vi "Main.vi"(11 "Module Admin":refnum<class "Delacor_lib_QMH_Module Admin.lvclass">) -> ()   [LabVIEW 2020, in "Acquisition.lvlib"]
doc: "This template is based off of the Queued Message Handler design pattern and the Queued Message Handler project template that ships with LabVIEW.\n\nThe main difference is that the queue is private to this module and communication between modules is performed via Broadcast and Request events.\n\nRequest events are wrapped in public API methods and are handled in the Event Handling Loop (EHL) of this VI. Any module can register for Broadcast events sent by this module. The EHL generates messages based on user interface actions.\n\nThe Message Handling Loop (MHL) processes messages generated by the EHL, or by other messages. The messages are string values, so new messages can be added easily to the Message Cases case structure in the MHL. Each message cluster can also provide an optional value for Message Data, which is a variant that can be converted to whatever message-specific data is required.\n_____\nBased on Delacor QMH Project Template 5.0.0.82."
uses:
  Acquisition.lvlib
  <vilib>/Delacor/Delacor QMH/Libraries/Module Admin_class/Delacor_lib_QMH_Module Admin.lvclass
  Module Data--cluster.ctl
  Stop Helper Loop Argument--cluster.ctl
  <vilib>/Delacor/Delacor QMH/Libraries/Message Queue_class/Delacor_lib_QMH_Message Queue.lvclass/Delacor_lib_QMH_Message Queue.ctl
  Stop Argument--cluster.ctl
  <vilib>/Delacor/Delacor QMH/Libraries/Module Admin_class/Delacor_lib_QMH_Module Admin.lvclass/Delacor_lib_QMH_Module Admin.ctl
  <vilib>/Utility/miscctls.llb/LVPointTypeDef.ctl
  <vilib>/Delacor/Delacor QMH/Libraries/Message Queue_class/Delacor_lib_QMH_Enqueue Message (Single).vi
  <vilib>/Delacor/Delacor QMH/Libraries/Module Admin_class/Delacor_lib_QMH_Get External Launch.vi
  <vilib>/Utility/error.llb/Error Cluster From Error Code.vi
  <vilib>/ErrorRing/Error Ring.xnode
  <vilib>/Delacor/Delacor QMH/Libraries/Message Queue_class/Delacor_lib_QMH_Message Queue.lvclass
panel:
  out "Time Stamp":timestamp
  in  "Simulate MHL Error":bool
  in  "Simulate EHL Error":bool
  out "error out":errorcluster
  out "Status":string
  # "Other QMH Modules communicate with this Module via its Public API (wrappers for its Request Events).\n\nThis Module communicates with other Modules via its Broadcast Events.\nAny module that wants to get these messages, just registers for this module's Broadcast events."
  # "This template is for the Delacor Modified Queued Message Handler design pattern.\n\nSee the block diagram for more information on how to use this template."
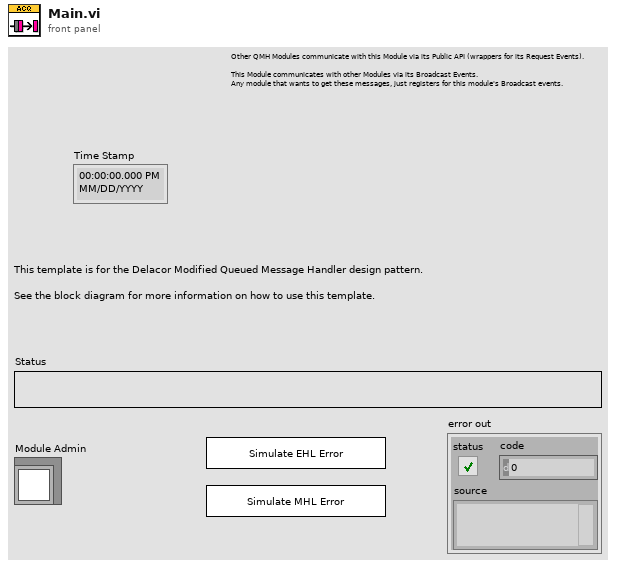
[diagram p1: front panel]
types:
  T1 = typedef "Acquisition.lvlib/Request Events--cluster.ctl" = cluster{"Stop Module":refnum<user-event>, "Show Panel":refnum<user-event>, "Hide Panel":refnum<user-event>, "Get Module Execution Status":refnum<user-event>, "Show Diagram":refnum<user-event>, "Start Helper Loop":refnum<user-event>, "Stop Helper Loop":refnum<user-event>}
  T2 = typedef "Acquisition.lvlib/Module Data--cluster.ctl" = cluster{"Status":string}
  T3 = enum32{"invalid lock state", "Not Locked", "Locked (No Password)", "Password-protected"}
  T4 = typedef "Acquisition.lvlib/Stop Argument--cluster.ctl" = cluster{"Origin":string, "Exit via Stop Module Req?":bool, "Wait for Module to stop?":bool}
  T5 = typedef "LVPointTypeDef.ctl" = cluster{"Horizontal":i16, "Vertical":i16}
  T6 = enum32{"Invalid", "Standard", "Closed", "Hidden", "Minimized", "Maximized"}
  T7 = typedef "Acquisition.lvlib/Stop Helper Loop Argument--cluster.ctl" = cluster{"Boolean":bool}
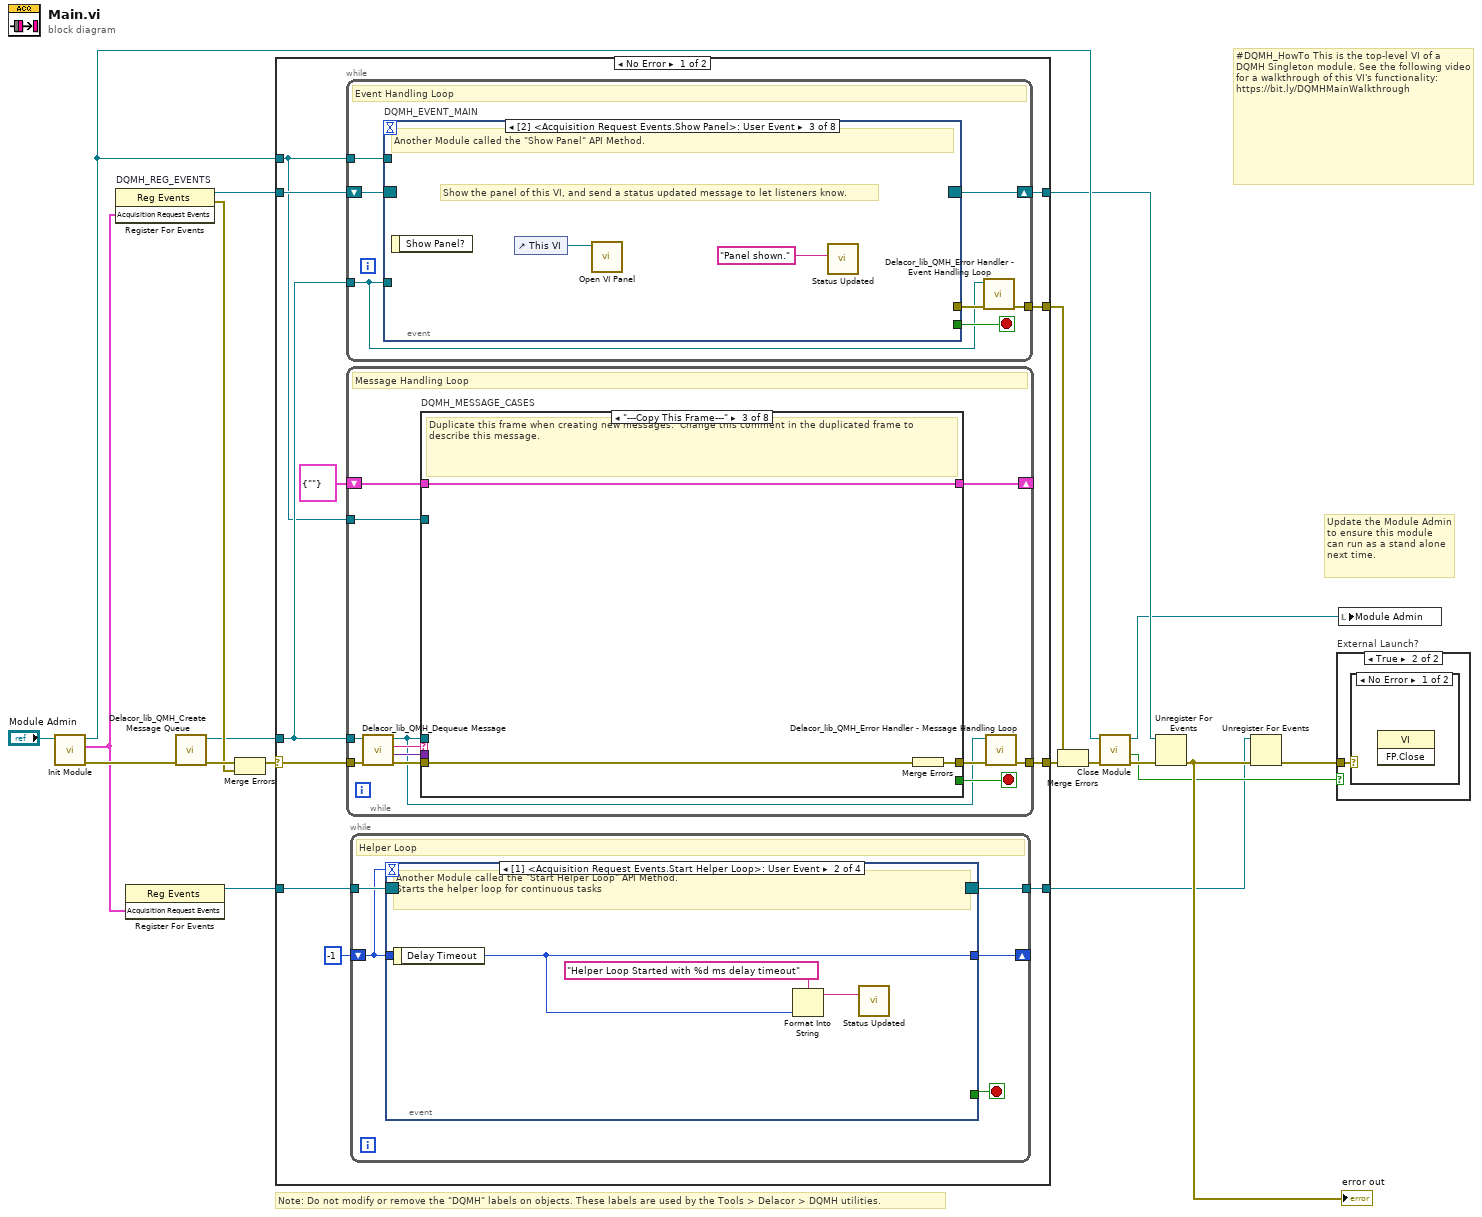
[diagram p0: block diagram]
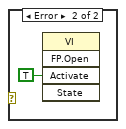
[diagram p3: hidden frame]
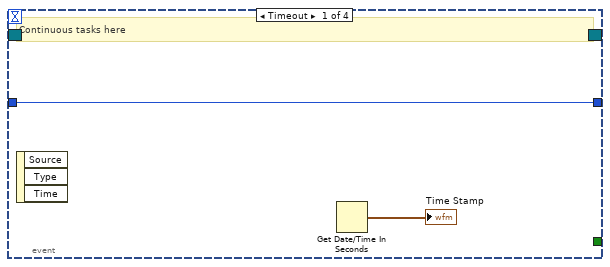
[diagram p4: hidden frame]
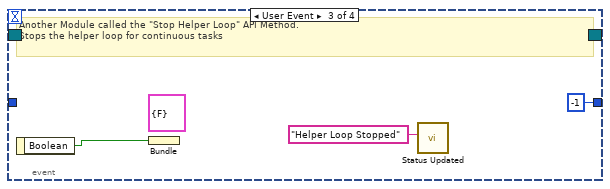
[diagram p5: hidden frame]
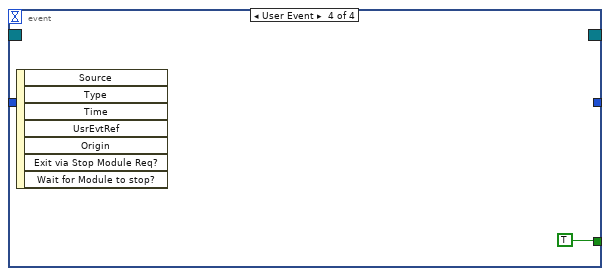
[diagram p6: hidden frame]
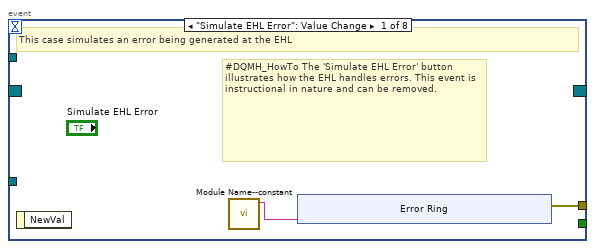
[diagram p7: hidden frame]
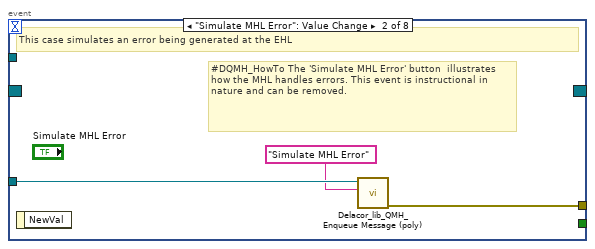
[diagram p8: hidden frame]
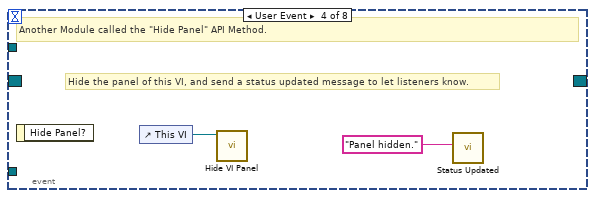
[diagram p9: hidden frame]
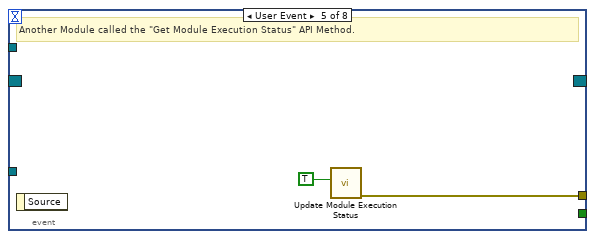
[diagram p10: hidden frame]
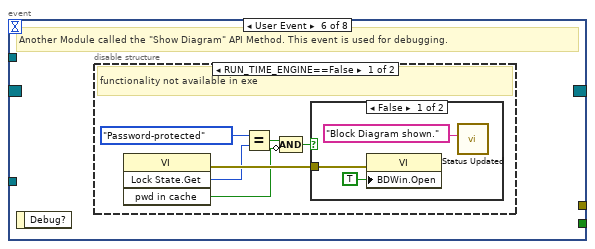
[diagram p11: hidden frame]
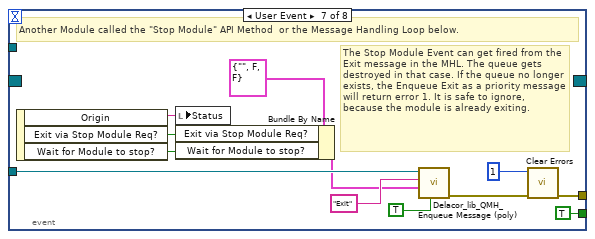
[diagram p14: hidden frame]
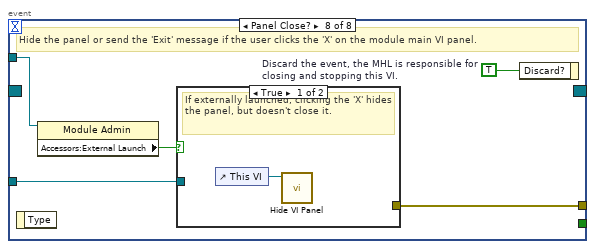
[diagram p15: hidden frame]
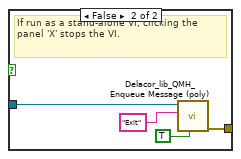
[diagram p16: hidden frame]
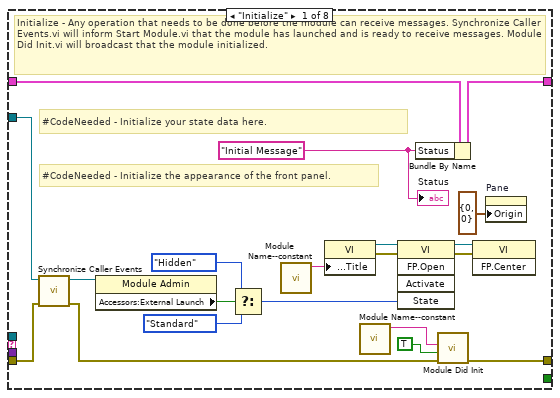
[diagram p17: hidden frame]
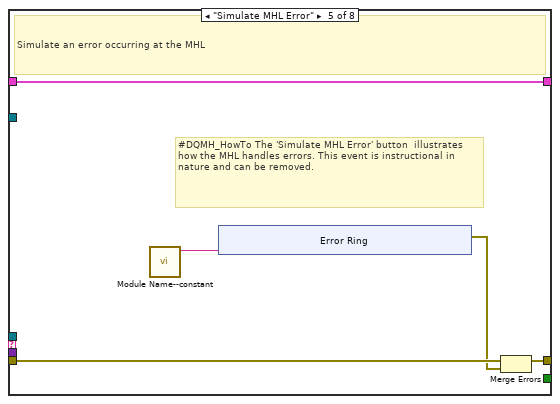
[diagram p20: hidden frame]
diagram:
  # "#DQMH_HowTo This is the top-level VI of a DQMH Singleton module. See the following video for a walkthrough of this VI's functionality: https://bit.ly/DQMHMainWalkthrough"
  # "Note: Do not modify or remove the \"DQMH\" labels on objects. These labels are used by the Tools > Delacor > DQMH utilities."
  # "Update the Module Admin to ensure this module can run as a stand alone next time."
  n1 = call "Init Module.vi"("Singleton Module Admin in"="Module Admin") -> ("error out"=w19:errorcluster, "Acquisition Request Events"=w3:T1, "Singleton Module Admin out"=w11:refnum<class "Delacor_lib_QMH_Module Admin.lvclass">)  [unwired: 8 in]
  n2 = register-events "DQMH_REG_EVENTS"(w3) -> (reference out=w9:refnum<event-registration>, error out=w12:errorcluster)  [unwired: 2 in]
  n3 = register-events(w3) -> (reference out=w4:refnum<event-registration>)  [unwired: 2 in, 1 out]
  n4 = call <vilib>:"Delacor_lib_QMH_Create Message Queue.vi"("error in (no error)"=w19) -> ("error out"=w14:errorcluster, "Message Queue"=w8:refnum<class "Delacor_lib_QMH_Message Queue.lvclass">)  [unwired: 9 in]
  n5 = Merge Errors(w14, w12) -> (w13:errorcluster)
  n6 = case shown="No Error" w13 {
    selector: w13 -> [w29 w202]
    tunnel: [w31 w201] -> w20
    tunnel: [w28 w207] -> w10
    tunnel: w9 -> [w26 w207]
    tunnel: w8 -> [w25 w200]
    tunnel: [w30 _] -> w17
    tunnel: w11 -> [w24 w203]
    tunnel: w4 -> [w23 w199]
    tunnel: [w22 w199] -> w1
    frame No Error {
      n7 = while {
        tunnel: w25 -> [w46]
        shift-right: [w49] -> w28
        shift-left: w26 -> [w50]
        tunnel: [w51] -> w30
        tunnel: w24 -> [w47]
        stop <- w48 stop-if-true
        # "Event Handling Loop"
        n8 = event "DQMH_EVENT_MAIN" shown="[2] <Acquisition Request Events.Show Panel>: User Event" {
          selector: w50 -> [_ _ _ _ _ _ _ _]
          dyn-events: [_ _ _ _ _ _ _ _] -> w49
          timeout: _ -> [_ _ _ _ _ _ _ _]
          tunnel: [_ _ _ _ _ _ TRUE ("Discard?") _] -> w48
          tunnel: w46 -> [_ w63 _ _ _ _ w87 w94]
          tunnel: [w54 w64 _ _ w70 _ w90 w96] -> w52
          tunnel: w47 -> [_ _ _ _ _ _ _ w93]
          event "Simulate EHL Error": Value Change {
            # "#DQMH_HowTo The 'Simulate EHL Error' button  illustrates how the EHL handles errors. This event is instructional in nature and can be removed."
            # "This case simulates an error being generated at the EHL"
            n9 = event-data() -> ()  [unwired: 1 in, 1 out]
            n10 = call "Module Name--constant.vi"() -> ("Module Name"=w53:string)  [unwired: 11 in]
            n11 = xnode "Error Ring"("parameter 0"=w53) -> ("error out"=w54:errorcluster)
          }
          event "Simulate MHL Error": Value Change {
            # "#DQMH_HowTo The 'Simulate MHL Error' button  illustrates how the MHL handles errors. This event is instructional in nature and can be removed."
            # "This case simulates an error being generated at the EHL"
            n12 = event-data() -> ()  [unwired: 1 in, 1 out]
            n13 = call-poly <vilib>:"Delacor_lib_QMH_Enqueue Message (poly).vi"("Message"="Simulate MHL Error", "Message Queue in"=w63) -> ("error out"=w64:errorcluster)  [unwired: 8 in, 1 out]
          }
          event User Event {
            # "Show the panel of this VI, and send a status updated message to let listeners know."
            # "Another Module called the \"Show Panel\" API Method."
            n14 = event-data() -> ()  [unwired: 1 in, 1 out]
            n15 = control-ref of="This VI"() -> (w66:refnum<vi>)
            n16 = call "Open VI Panel.vi"("VI"=w66) -> ()  [unwired: 10 in, 1 out]
            n17 = call "Status Updated.vi"("Status"="Panel shown." ("format string")) -> ()  [unwired: 10 in, 1 out]
          }
          event User Event {
            # "Hide the panel of this VI, and send a status updated message to let listeners know."
            # "Another Module called the \"Hide Panel\" API Method."
            n18 = event-data() -> ()  [unwired: 1 in, 1 out]
            n19 = control-ref of="This VI"() -> (w68:refnum<vi>)
            n20 = call "Hide VI Panel.vi"("VI"=w68) -> ()  [unwired: 10 in, 1 out]
            n21 = call "Status Updated.vi"("Status"="Panel hidden." ("format string")) -> ()  [unwired: 10 in, 1 out]
          }
          event User Event {
            # "Another Module called the \"Get Module Execution Status\" API Method."
            n22 = event-data() -> ()  [unwired: 1 in, 1 out]
            n23 = call "Update Module Execution Status.vi"("Running?"=TRUE) -> ("error out"=w70:errorcluster)  [unwired: 10 in]
          }
          event User Event {
            # "Another Module called the \"Show Diagram\" API Method. This event is used for debugging."
            n24 = event-data() -> ()  [unwired: 1 in, 1 out]
            n25 = disable-structure shown="RUN_TIME_ENGINE==False" {
              frame condition #0 (active) {
                # "functionality not available in exe"
                n26 = invoke class="VI" method="Lock State.Get"() -> (error out=w76:errorcluster, "Get Lock State"=w75:T3, "pwd in cache"=w72:bool)  [unwired: 4 in, 1 out]
                n27 = Equal?(x=T3."Password-protected", y=w75) -> (x = y?=w73:bool)
                n28 = Compound Arithmetic op=AND(w73, invert w72) -> (w71:bool)
                n29 = case shown="False" w71 {
                  tunnel: w76 -> [w79 _]
                  frame False {
                    n30 = property class="VI"(error in=w79, "BDWin.Open"=TRUE ("Block Diagram Window:Open")) -> ()  [unwired: 1 in, 2 out]
                    n31 = call "Status Updated.vi"("Status"="Block Diagram shown." ("format string")) -> ()  [unwired: 10 in, 1 out]
                  }
                  frame True {
                    # "Password-protected VI, and the password is not in the cache. Do not show the diagram."
                  }
                }
              }
              frame condition #1 {
              }
            }
          }
          event User Event {
            # "The Stop Module Event can get fired from the Exit message in the MHL. The queue gets destroyed in that case. If the queue no longer exists, the Enqueue Exit as a priority message will return error 1. It is safe to ignore, because the module is already exiting."
            # "Another Module called the \"Stop Module\" API Method  or the Message Handling Loop below."
            n32 = event-data() -> ("Origin"=w86:string, "Exit via Stop Module Req?"=w82:bool, "Wait for Module to stop?"=w81:bool)  [unwired: 1 in]
            n33 = local write "Status"(w86) -> ()
            n34 = Bundle By Name(cluster=T4 {"Origin"="", "Exit via Stop Module Req?"=FALSE, "Wait for Module to stop?"=FALSE} ("Stop Argument"), "Exit via Stop Module Req?"=w82, "Wait for Module to stop?"=w81) -> (w80:T4)
            n35 = call-poly <vilib>:"Delacor_lib_QMH_Enqueue Message (poly).vi"("Priority Message? (F)"=TRUE, "Message Data"=w80, "Message"="Exit", "Message Queue in"=w87) -> ("error out"=w91:errorcluster)  [unwired: 6 in, 1 out]
            n36 = call <vilib>:"Clear Errors.vi"("error in (no error)"=w91, "specific error code to clear (0: all)"=1) -> ("error out"=w90:errorcluster)  [unwired: 4 in, 1 out]
          }
          event Panel Close? {
            w95 = TRUE  # Discard the event, the MHL is responsible for closing and stopping this VI.
            # "Hide the panel or send the 'Exit' message if the user clicks the 'X' on the module main VI panel."
            n37 = event-data() -> ()  [unwired: 1 in, 1 out]
            n38 = property class="Module Admin"(reference=w93) -> ("Accessors:External Launch"=w92:bool)  [unwired: 1 in, 2 out]
            n39 = case shown="True" w92 {
              tunnel: w94 -> [_ w100]
              tunnel: [_ w101] -> w96
              frame True {
                # "If externally launched, clicking the 'X' hides the panel, but doesn't close it."
                n40 = control-ref of="This VI"() -> (w97:refnum<vi>)
                n41 = call "Hide VI Panel.vi"("VI"=w97) -> ()  [unwired: 10 in, 1 out]
              }
              frame False {
                # "If run as a stand-alone VI, clicking the panel 'X' stops the VI."
                n42 = call-poly <vilib>:"Delacor_lib_QMH_Enqueue Message (poly).vi"("Priority Message? (F)"=TRUE, "Message"="Exit", "Message Queue in"=w100) -> ("error out"=w101:errorcluster)  [unwired: 7 in, 1 out]
              }
            }
            n43 = event-data("Discard?"=w95) -> ()  [unwired: 1 in, 1 out]
          }
        }
        n44 = call-dynamic "Delacor_lib_QMH_Error Handler - Event Handling Loop.vi"("error in (no error)"=w52, "Message Queue in"=w46) -> ("dup error in"=w51:errorcluster)  [unwired: 8 in, 1 out]
      }
      n45 = while {
        tunnel: w25 -> [w104]
        shift-right: [w108] -> _
        shift-left: T2 {"Status"=""} ("Data Cluster") -> [w109]
        tunnel: w29 -> [w112]
        tunnel: [w110] -> w31
        tunnel: w24 -> [w102]
        stop <- w107 stop-if-true
        # "Message Handling Loop"
        n46 = call-dynamic "Delacor_lib_QMH_Dequeue Message.vi"("error in (no error)"=w112, "Message Queue in"=w104) -> ("error out"=w111:errorcluster, "Message Data"=w105:variant, "Message"=w106:string, "Message Queue out"=w103:refnum<class "Delacor_lib_QMH_Message Queue.lvclass">)  [unwired: 6 in]
        n47 = case "DQMH_MESSAGE_CASES" shown="\"---Copy This Frame---\"" w106 {
          selector: w106 -> [_ _ _ _ _ _ _ w186]
          tunnel: w103 -> [_ _ _ _ _ w156 w178 _]
          tunnel: w111 -> [w131 w135 w138 w140 w145 w163 w184 w188]
          tunnel: [w129 w135 w137 w140 w144 w159 w181 w189] -> w113
          tunnel: w109 -> [w120 w134 w136 w139 w142 w158 w177 w187]
          tunnel: [w119 w134 w136 w139 w142 w158 w177 w187] -> w108
          tunnel: [_ _ _ _ _ _ w176 _] -> w107
          tunnel: w105 -> [_ _ _ _ _ w157 w175 _]
          tunnel: w102 -> [w121 _ _ _ _ w155 w170 _]
          frame "Initialize" {
            w114 = "Initial Message" ("Initial Message")
            # "#CodeNeeded - Initialize the appearance of the front panel."
            # "#CodeNeeded - Initialize your state data here."
            # "Initialize - Any operation that needs to be done before the module can receive messages. Synchronize Caller Events.vi will inform Start Module.vi that the module has launched and is ready to receive messages. Module Did Init.vi will broadcast that the module initialized."
            n48 = call "Synchronize Caller Events.vi"("error in (no error)"=w131, "Singleton Module Admin in"=w121) -> ("error out"=w130:errorcluster, "Singleton Module Admin out"=w116:refnum<class "Delacor_lib_QMH_Module Admin.lvclass">)  [unwired: 8 in]
            n49 = property class="Module Admin"(reference=w116) -> ("Accessors:External Launch"=w125:bool)  [unwired: 1 in, 2 out]
            n50 = Select(t=T6."Hidden" ("State"), s=w125, f=T6."Standard" ("State")) -> (s? t:f=w122:T6)
            n51 = call "Module Name--constant.vi"() -> ("Module Name"=w128:string)  [unwired: 11 in]
            n52 = property class="VI"("Front Panel.Title"=w128) -> (reference out=w127:refnum<vi>, error out=w133:errorcluster)  [unwired: 2 in]
            n53 = call "Module Name--constant.vi"() -> ("Module Name"=w117:string)  [unwired: 11 in]
            n54 = invoke class="VI" method="FP.Open"(reference=w127, error in=w133, "State"=w122) -> (reference out=w126:refnum<vi>, error out=w132:errorcluster)  [unwired: 2 in, 3 out]
            n55 = Bundle By Name(cluster=w120, "Status"=w114) -> (w119:T2)
            n56 = call "Module Did Init.vi"("error in (no error)"=w130, "Initialized?"=TRUE, "Origin"=w117) -> ("error out"=w129:errorcluster)  [unwired: 8 in]
            n57 = invoke class="VI" method="FP.Center"(reference=w126, error in=w132) -> ()  [unwired: 1 in, 3 out]
            n58 = property on="Pane" class="Pane"("Origin"=T5 {"Horizontal"=0, "Vertical"=0}) -> ()  [unwired: 2 in, 2 out]
            "Status" <- w114
          }
          frame "--- Module Specific ---" {
            # "Separator -- The following cases handle messages specific to this Module."
          }
          frame "---Copy This Frame---" {
            # "Duplicate this frame when creating new messages.  Change this comment in the duplicated frame to describe this message."
            n59 = Merge Errors(w138) -> (w137:errorcluster)
          }
          frame "--- Exit and Error Handling---" {
            # "Separator - The following cases handle errors and exit messages."
          }
          frame "Simulate MHL Error" {
            # "#DQMH_HowTo The 'Simulate MHL Error' button  illustrates how the MHL handles errors. This event is instructional in nature and can be removed."
            # "Simulate an error occurring at the MHL"
            n60 = call "Module Name--constant.vi"() -> ("Module Name"=w141:string)  [unwired: 11 in]
            n61 = xnode "Error Ring"("parameter 0"=w141) -> ("error out"=w143:errorcluster)
            n62 = Merge Errors(w145, w143) -> (w144:errorcluster)
          }
          frame "Error" {
            # "#CodeRecommended - If you ever change the name of this \"Error\" message, you'll need to update the name in the Check Loop Error.vi as well."
            # "#CodeRecommended - If the module is running in standalone mode (External Launch = FALSE), this code will pop up an error dialog and call the 'Exit' message if an error occurs. Add more fine-grained error handling here."
            # "Error - Check the error message data and respond accordingly. This message is sent by the \"Error Handler\" VIs at the end of each loop in this application."
            n63 = property class="Module Admin"(reference=w155) -> ("Accessors:External Launch"=w154:bool)  [unwired: 1 in, 2 out]
            n64 = Variant To Data(error in=w163, type=errorcluster {"status"=FALSE, "code"=0, "source"=""} ("error constant"), Variant=w157) -> (data=w164:errorcluster, error out=w161:errorcluster)
            n65 = call "Module Name--constant.vi"() -> ("Module Name"=w153:string)  [unwired: 11 in]
            n66 = call "Error Reported.vi"("Additional Information"=w153, "Error"=w164) -> ()  [unwired: 9 in, 1 out]
            n67 = case shown="False" w154 {
              tunnel: [w169 _] -> w160
              tunnel: w156 -> [w167 _]
              tunnel: w164 -> [w168 _]
              frame False {
                # "If the module is running standalone, then pop up an error dialog and call the \"Exit\" message."
                n68 = call <vilib>:"Simple Error Handler.vi"("error in (no error)"=w168) -> ()  [unwired: 4 in, 5 out]
                n69 = call-poly <vilib>:"Delacor_lib_QMH_Enqueue Message (poly).vi"("Priority Message? (F)"=TRUE, "Message"="Exit", "Message Queue in"=w167) -> ("error out"=w169:errorcluster)  [unwired: 7 in, 1 out]
              }
              frame True {
                # "If the module was launched externally, calling the Error Reported broadcast VI is the only action performed by the \"Error\" message. The module's caller can then process the error appropriately."
              }
            }
            n70 = Merge Errors(w161, w160) -> (w159:errorcluster)
            n71 = local write "error out"(w159) -> ()
          }
          frame "Exit" {
            w174 = 91  # 91: not all Exit messages will have an argument
            w176 = TRUE  # Stop the VI
            # "Release the message queue reference"
            # "#CodeNeeded - Add any required cleanup code here"
            # "Exit - Exit the application."
            n72 = Variant To Data(error in=w184, type=T4 {"Origin"="", "Exit via Stop Module Req?"=FALSE, "Wait for Module to stop?"=FALSE} ("Stop Argument"), Variant=w175) -> (data=w172:T4, error out=w180:errorcluster)
            n73 = call <vilib>:"Clear Errors.vi"("error in (no error)"=w180, "specific error code to clear (0: all)"=w174) -> ("error out"=w183:errorcluster)  [unwired: 4 in, 1 out]
            n74 = control-ref of="This VI"() -> (w171:refnum<vi>)
            n75 = call-dynamic "Delacor_lib_QMH_Release Message Queue.vi"("error in (no error)"=w183, "Message Queue"=w178) -> ("error out"=w182:errorcluster)  [unwired: 9 in]
            n76 = call "Handle Exit.vi"("Stop Argument"=w172, "Admin in"=w170, "VI reference"=w171) -> ("error out"=w179:errorcluster)  [unwired: 7 in, 1 out]
            n77 = Merge Errors(w182, w179) -> (w181:errorcluster)
          }
          frame Default {
            # "'Default' case only runs if there is a message that isn't defined in any of the other cases.  Output a programming error."
            n78 = call "Module Name--constant.vi"() -> ("Module Name"=w185:string)  [unwired: 11 in]
            n79 = xnode "Error Ring"("parameter 0"=w186, "parameter 1"=w185) -> ("error out"=w190:errorcluster)
            n80 = Merge Errors(w188, w190) -> (w189:errorcluster)
          }
        }
        n81 = call-dynamic "Delacor_lib_QMH_Error Handler - Message Handling Loop.vi"("error in (no error)"=w113, "Message Queue in"=w103) -> ("dup error in"=w110:errorcluster)  [unwired: 8 in, 1 out]
      }
      n82 = while {
        tunnel: w23 -> [w36]
        tunnel: [w35] -> w22
        shift-right: [w33] -> _
        shift-left: -1 -> [w32]
        stop <- w34 stop-if-true
        # "Helper Loop"
        n83 = event shown="[1] <Acquisition Request Events.Start Helper Loop>: User Event" {
          selector: w36 -> [_ _ _ _]
          dyn-events: [_ _ _ _] -> w35
          timeout: w32 -> [_ _ _ _]
          tunnel: [_ _ _ TRUE] -> w34
          tunnel: [w38 w41 -1 _] -> w33
          tunnel: w32 -> [w38 _ _ _]
          event Timeout {
            # "Continuous tasks here"
            n84 = event-data() -> ()  [unwired: 1 in, 3 out]
            n85 = Get Date/Time In Seconds() -> (seconds since 1Jan1904=→"Time Stamp":timestamp)
          }
          event User Event {
            # "Another Module called the \"Start Helper Loop\" API Method.\nStarts the helper loop for continuous tasks"
            n86 = event-data() -> ("Delay Timeout"=w41:i32)  [unwired: 1 in]
            n87 = Format Into String(format string="Helper Loop Started with %d ms delay timeout", w41) -> (resulting string=w40:string)  [unwired: 2 in, 1 out]
            n88 = call "Status Updated.vi"("Status"=w40) -> ()  [unwired: 10 in, 1 out]
          }
          event User Event {
            (unwired) T7 {"Boolean"=FALSE} ("Stop Helper Loop Argument")
            # "Another Module called the \"Stop Helper Loop\" API Method.\nStops the helper loop for continuous tasks"
            n89 = event-data() -> ("Boolean"=w44:bool)  [unwired: 1 in]
            n90 = Bundle("Boolean"=w44) -> ()  [unwired: 1 in, 1 out]
            n91 = call "Status Updated.vi"("Status"="Helper Loop Stopped") -> ()  [unwired: 10 in, 1 out]
          }
          event User Event {
            n92 = event-data() -> ()  [unwired: 1 in, 7 out]
          }
        }
      }
    }
    frame Error {
      # "Synchronize Caller Events.vi will inform Start Module.vi that the module has launched and will let the code calling Start Module.vi register for broadcasts and would permit the caller receive the broadcast that an error occurred at launch time."
      n93 = call-dynamic "Delacor_lib_QMH_Release Message Queue.vi"("error in (no error)"=w202, "Message Queue"=w200) -> ("error out"=w201:errorcluster)  [unwired: 9 in]
      n94 = call "Synchronize Caller Events.vi"("Singleton Module Admin in"=w203) -> ("error out"=w208:errorcluster)  [unwired: 9 in, 1 out]
      n95 = call "Module Name--constant.vi"() -> ("Module Name"=w206:string)  [unwired: 11 in]
      n96 = Format Into String(format string="An error occurred during initialization. %s is no longer running.", w206) -> (resulting string=w204:string)  [unwired: 2 in, 1 out]
      n97 = Merge Errors(w201, w208) -> (w209:errorcluster)
      n98 = call "Error Reported.vi"("Additional Information"=w204, "Error"=w209) -> ()  [unwired: 9 in, 1 out]
    }
  }
  n99 = Merge Errors(w17, w20) -> (w16:errorcluster)
  n100 = call "Close Module.vi"("error in (no error)"=w16, "Module Admin in"=w11) -> ("error out"=w18:errorcluster, "External Launch"=w5:bool, "Module Admin out"=w6:refnum<class "Delacor_lib_QMH_Module Admin.lvclass">)  [unwired: 7 in]
  n101 = Unregister For Events(event registration refnum=w10, error in=w18) -> (error out=w15:errorcluster)
  "error out" <- w15
  n102 = Unregister For Events(event registration refnum=w1, error in=w15) -> (error out=w2:errorcluster)
  n103 = case "External Launch?" shown="True" w5 {
    tunnel: w2 -> [_ w210]
    frame False {
    }
    frame True {
      n104 = case shown="No Error" w210 {
        frame No Error {
          n105 = invoke class="VI" method="FP.Close"() -> ()  [unwired: 3 in, 3 out]
        }
        frame Error {
          n106 = invoke class="VI" method="FP.Open"("Activate"=TRUE ("Activate?")) -> ()  [unwired: 4 in, 5 out]
        }
      }
    }
  }
  n107 = local write "Module Admin"(w6) -> ()
